vi "Setup2182-2400.vi"() -> ()   [LabVIEW 2020]
panel:
  in  "Delay":dbl=0.02
  in  "2400 CURR":dbl=1.0
  in  "2400 GPIB add":string="23"
  in  "2182 GPIB add":string="22"
  # "Ultra Low Resistance - Delta Mode Measurements using 2400 and 2182."
  # "KEITHLEY"
  # "Connect Trigger Link Cable between 2182 & 2400.\nNote that moving average (digital) filter is on by default,\navg = 10rdgs, window = 0.01%"
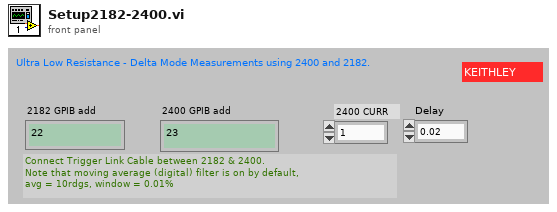
[diagram p1: front panel]
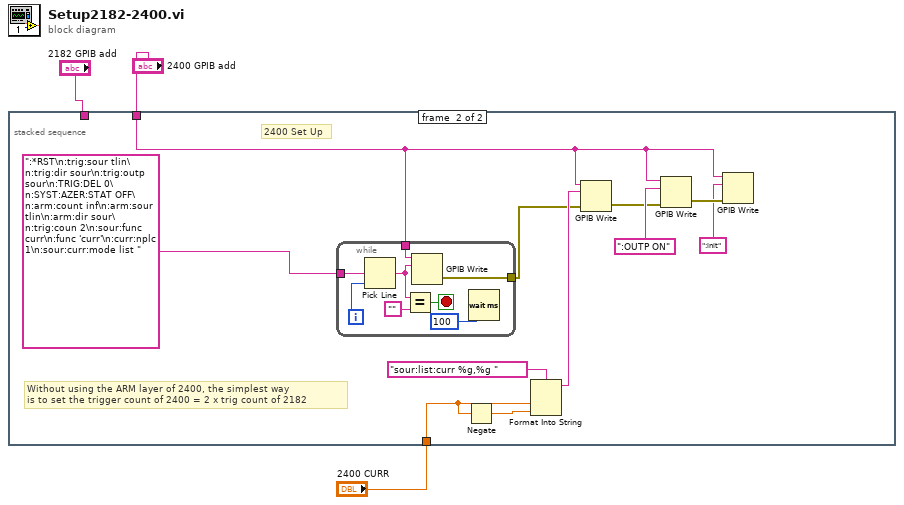
[diagram p0: block diagram]
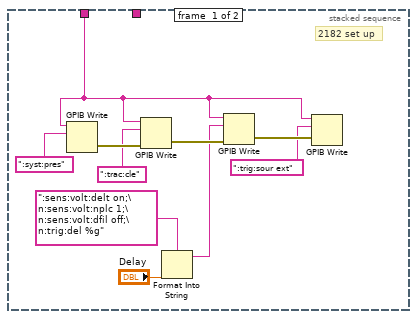
[diagram p2: hidden frame]
diagram:
  n1 = stacked-sequence {
    tunnel: "2182 GPIB add" -> [w8 _]
    tunnel: "2400 GPIB add" -> [_ w14]
    tunnel: "2400 CURR" -> [_ w21]
    frame #0 {
      # "2182 set up"
      n2 = GPIB Write(0:w8, 1:":syst:pres") -> (6:w13:errorcluster)  [unwired: 3 in, 1 out]
      n3 = GPIB Write(0:w8, 1:":trac:cle", 3:w13) -> (6:w7:errorcluster)  [unwired: 2 in, 1 out]
      n4 = Format Into String(format string=":sens:volt:delt on;\n:sens:volt:nplc 1;\n:sens:volt:dfil off;\n:trig:del %g", "Delay") -> (resulting string=w4:string)  [unwired: 2 in, 1 out]
      n5 = GPIB Write(0:w8, 1:w4, 3:w7) -> (6:w10:errorcluster)  [unwired: 2 in, 1 out]
      n6 = GPIB Write(0:w8, 1:":trig:sour ext", 3:w10) -> ()  [unwired: 2 in, 2 out]
    }
    frame #1 {
      # "Without using the ARM layer of 2400, the simplest way\nis to set the trigger count of 2400 = 2 x trig count of 2182"
      # "2400 Set Up"
      n7 = while {
        tunnel: ":*RST\n:trig:sour tlin\n:trig:dir sour\n:trig:outp sour\n:TRIG:DEL 0\n:SYST:AZER:STAT OFF\n:arm:count inf\n:arm:sour tlin\n:arm:dir sour\n:trig:coun 2\n:sour:func curr\n:func 'curr'\n:curr:nplc 1\n:sour:curr:mode list " -> [w31]
        tunnel: [w27] -> w20
        tunnel: w14 -> [w26]
        i -> [w32]
        stop <- w30 stop-if-true
        n8 = Pick Line(multi-line string=w31, line index=w32) -> (output string=w28:string)  [unwired: 1 in]
        n9 = Equal?(x=w28, y="") -> (x = y?=w30:bool)
        n10 = GPIB Write(0:w26, 1:w28) -> (6:w27:errorcluster)  [unwired: 3 in, 1 out]
        n11 = Wait (ms)(milliseconds to wait=u32 100) -> ()  [unwired: 1 out]
      }
      n12 = Negate(x=w21) -> (-x=w24:dbl)
      n13 = Format Into String(format string="sour:list:curr %g,%g ", w21, w24) -> (resulting string=w23:string)  [unwired: 2 in, 1 out]
      n14 = GPIB Write(0:w14, 1:w23, 3:w20) -> (6:w15:errorcluster)  [unwired: 2 in, 1 out]
      n15 = GPIB Write(0:w14, 1:":OUTP ON", 3:w15) -> (6:w18:errorcluster)  [unwired: 2 in, 1 out]
      n16 = GPIB Write(0:w14, 1:":init", 3:w18) -> ()  [unwired: 2 in, 2 out]
    }
  }
